vi "Get SMO Public API.vi"(8 "error in (no error)":errorcluster, 11 "instrument.PPMS2 in":refnum<class "instrument.PPMS2.lvclass">) -> (0 "error out":errorcluster, 2 "Commands":string[](array[string]), 3 "instrument.PPMS2 out":refnum<class "instrument.PPMS2.lvclass">)   [LabVIEW 2019, in "instrument.PPMS2.lvclass"]
uses:
  instrument.PPMS2.lvclass
  instrument.PPMS/instrument.PPMS.lvclass
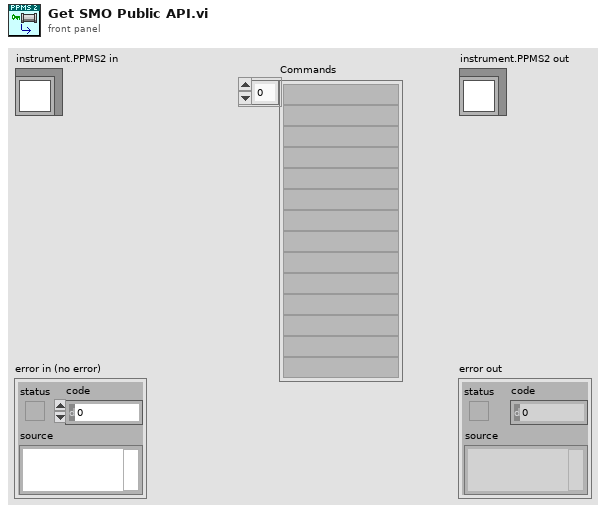
[diagram p1: front panel]
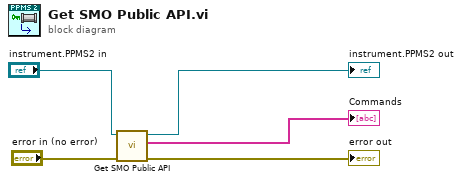
[diagram p0: block diagram]
diagram:
  n1 = call-parent "Get SMO Public API.vi"("error in (no error)"="error in (no error)", "instrument.PPMS in"="instrument.PPMS2 in") -> ("error out"=→"error out":errorcluster, "Commands"=→"Commands":string[], "instrument.PPMS out"=→"instrument.PPMS2 out":refnum<class "instrument.PPMS2.lvclass">)  [unwired: 7 in]
